vi "Read NMEA GPS GENERIC - no error - SubVI.vi"(0 "VISA resource name":refnum<visa-resource-name>="COM11", 5 "timeout (ms)":u32=10000, 7 "UTC Time Zone":i32=-5, 9 "stop":bool, 11 "error in (no error)":errorcluster, 12 "Baud Rate":dbl) -> (4 "GPS $GPRMC Data":T1 {"Course over ground (degrees)" format="%#.6g"; "Speed over ground (knots)" format="%#.6g"; "Magnetic Variation (degrees)" format="%#.6g"; "Longitude (ddmm.mmmm)" format="%#.6g"; "Lattitude (ddmm.mmmm)" format="%#.6g"}, 6 "GPS Data Valid?":bool, 10 "Stopped?":bool, 15 "error out":errorcluster)   [LabVIEW 2021]
doc: "This subVI decodes the most common NMEA-0183 sentence transmitted by GPS receivers, the $GPRMC sentence. The subvi returns time, position, ground speed, and magnetic variation. In the GPS interface configuration, use the \"NMEA OUT\" setting and set the baud rate to the standard 4800 bps setting. Connected to the computer's serial port using a PC Interface Cable, available from the GPS vendor. This subvi initializes the serial port on first call. On subsequent calls, the initialization is skipped. Always use the Stop input when stopping the VI so that the serial port connection is closed."
uses:
  <vilib>/Instr/_visa.llb/VISA Configure Serial Port (Instr).vi
panel:
  out "error out 2":errorcluster
  in  "Cluster":T1 {"Course over ground (degrees)" format="%_4g"; "Speed over ground (knots)" format="%_3g"; "Magnetic Variation (degrees)" format="%_4g"; "Longitude (ddmm.mmmm)" format="%_8g"; "Lattitude (ddmm.mmmm)" format="%_8g"}
  out "Variation\nEast/West":string
  out "Magnetic Variation \n(degrees)":dbl format="%_4g"
  out "Course over\nground (degrees)":dbl format="%_4g"
  out "Speed over \nground (knots)":dbl format="%_3g"
  out "Longitude\nEast/West":string
  out "Longitude\n(ddmm.mmmm)":dbl format="%_8g"
  out "Lattitude\nNorth/South":string
  out "Lattitude\n(ddmm.mmmm)":dbl format="%_8g"
  out "Local Time":timestamp
  out "UTC Time":timestamp
  in  "date time rec":T2
  out "Bytes read":u32
  out "String Read":string="\n"
  # "This subVI decodes the most common NMEA-0183 sentence transmitted by GPS receivers, the $GPRMC sentence. The subvi returns time, position, ground speed, and magnetic variation. In the GPS interface configuration, use the \"NMEA OUT\" setting and set the baud rate to the standard 4800 bps setting. Connected to the computer's serial port using a PC Interface Cable, available from the GPS vendor. This subvi initializes the serial port on first call. On subsequent calls, the initialization is skipped. Always use the Stop input when stopping the VI so that the serial port connection is closed."
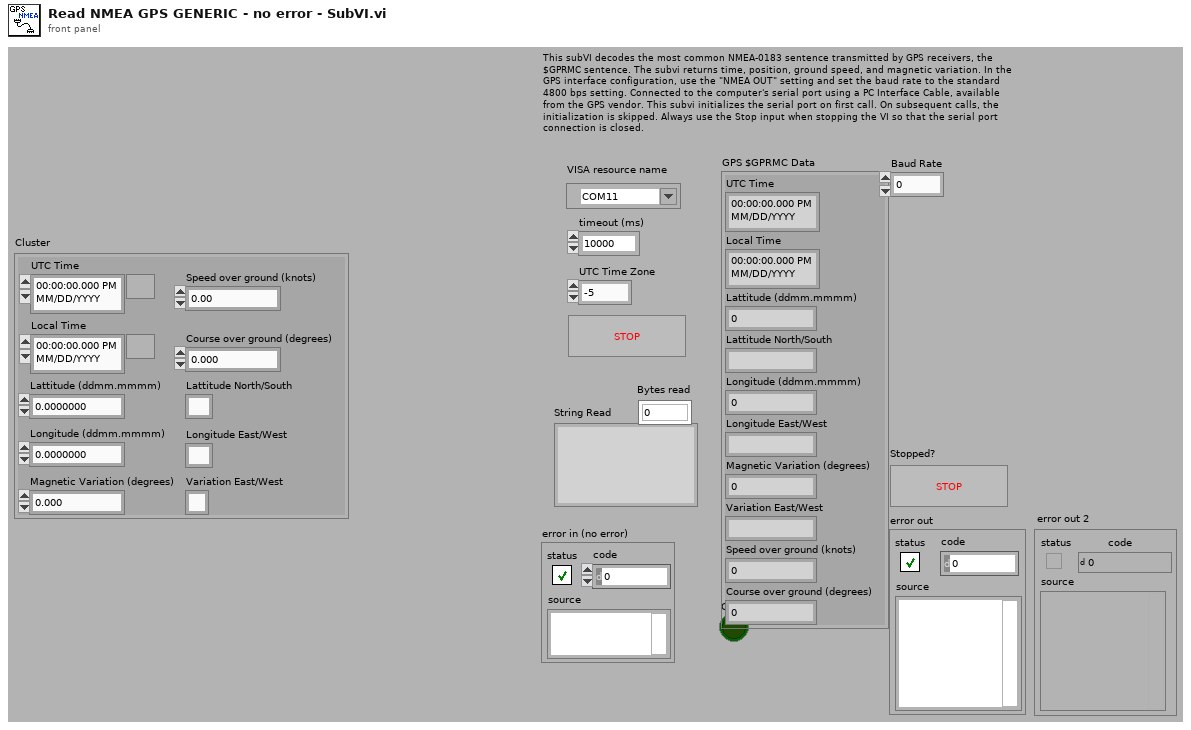
[diagram p1: front panel]
types:
  T1 = cluster{"UTC Time":timestamp, "Local Time":timestamp, "Lattitude (ddmm.mmmm)":dbl, "Lattitude North/South":string, "Longitude (ddmm.mmmm)":dbl, "Longitude East/West":string, "Magnetic Variation (degrees)":dbl, "Variation East/West":string, "Speed over ground (knots)":dbl, "Course over ground (degrees)":dbl}
  T2 = cluster{"second":i32, "minute":i32, "hour":i32, "day of month":i32, "month":i32, "year":i32, "day of week":i32, "day of year":i32, "is DST":i32}
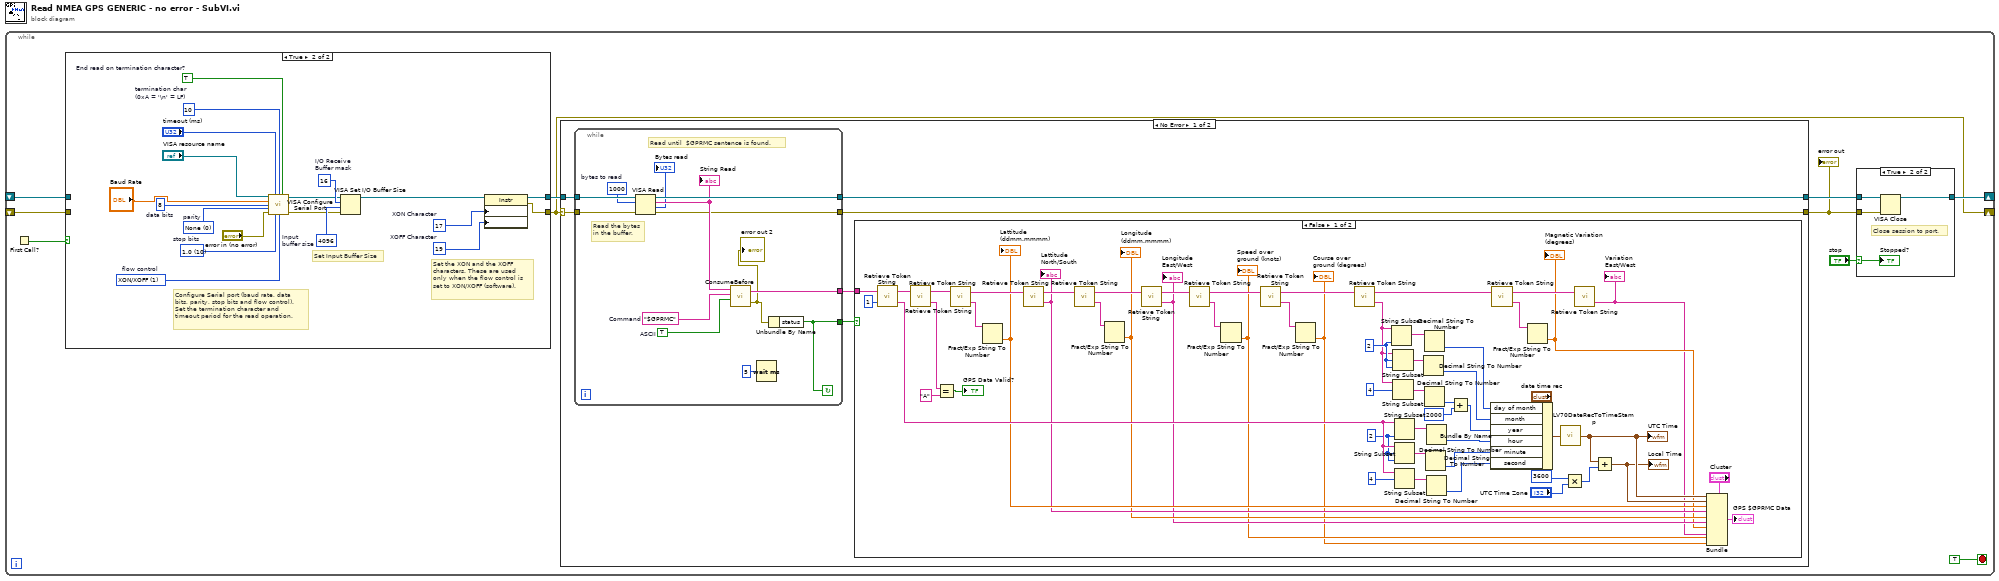
[diagram p0: block diagram]
diagram:
  n1 = while {
    shift-right: [w5] -> _
    shift-left: _ -> [w4]
    shift-right: [w3] -> _
    shift-left: _ -> [w2]
    stop <- TRUE stop-if-true
    n2 = First Call?() -> (First Call?: T/F=w8:bool)
    n3 = case shown="True" w8 {
      tunnel: [w16 w22] -> w10
      tunnel: [w15 w19] -> w3
      tunnel: w4 -> [w16 _]
      tunnel: w2 -> [w15 _]
      frame False {
      }
      frame True {
        w31 = TRUE  # End read on termination character?
        w24 = u8 19  # XOFF Character
        w25 = u8 17  # XON Character
        w29 = u32 4096  # Input buffer size
        w27 = u16 1 items=["None"=0, "XON/XOFF"=1, "RTS/CTS"=2, "DTR/DSR"=4]  # flow control
        w33 = u16 10 items=["1.0"=10, "1.5"=15, "2.0"=20]  # stop bits
        w34 = u16 0 items=["None", "Odd", "Even", "Mark", "Space"]  # parity
        w23 = u16 8  # data bits
        w28 = u8 10  # termination char (0xA = '\n' = LF)
        w30 = u16 16  # I/O Receive Buffer mask
        # "Set the XON and the XOFF\ncharacters. These are used\nonly when the flow control is\nset to XON/XOFF (software)."
        # "Configure Serial port (baud rate, data\nbits, parity, stop bits and flow control).\nSet the termination character and\ntimeout period for the read operation."
        # "Set Input Buffer Size"
        n4 = call-poly "VISA Configure Serial Port"("VISA resource name"="VISA resource name", "timeout (10sec)"="timeout (ms)", "termination char\n(0xA = '\\n' = LF)"=w28, "Enable Termination\nChar (T)"=w31, "baud rate (9600)"="Baud Rate", "data bits (8)"=w23, "parity (0:none)"=w34, "error in (no error)"="error in (no error)", "stop bits (10: 1 bit)"=w33, "flow control (0:none)"=w27) -> ("VISA resource name out"=w21:refnum<visa-resource-name>, "error out"=w20:errorcluster)  [unwired: 4 in]
        n5 = VISA Set I/O Buffer Size(VISA resource name=w21, mask (16)=w30, size (4096)=w29, error in (no error)=w20) -> (VISA resource name out=w26:refnum<visa-resource-name>)  [unwired: 1 out]
        n6 = property class="Instr"(reference=w26, "Serial Settings:Flow Control XON Character"=w25, "Serial Settings:Flow Control XOFF Character"=w24) -> (reference out=w22:refnum<visa-resource-name>, error out=w19:errorcluster)  [unwired: 1 in]
      }
    }
    n7 = case shown="No Error" w3 {
      selector: w3 -> [w39 w112]
      tunnel: w10 -> [w41 w113]
      tunnel: [w40 w113] -> w9
      tunnel: [w36 w112] -> w1
      frame No Error {
        n8 = while {
          tunnel: w41 -> [w54]
          tunnel: [w53] -> w40
          tunnel: [w43] -> w36
          tunnel: w39 -> [w52]
          tunnel: [w48] -> w38
          tunnel: [w45] -> w37
          stop <- w45 continue-if-true
          w47 = u32 1000  # bytes to read
          w51 = "$GPRMC"  # Command
          w50 = TRUE  # ASCII
          # "Read until  $GPRMC sentence is found."
          # "Read the bytes\nin the buffer."
          n9 = VISA Read(VISA resource name=w54, byte count=w47, error in (no error)=w52) -> (VISA resource name out=w53:refnum<visa-resource-name>, read buffer=w49:string, return count=→"Bytes read":u32, error out=w43:errorcluster)
          "String Read" <- w49
          n10 = call "ConsumeBefore.vi"("ASCII"=w50, "Before"=w51, "Response String In"=w49) -> ("error out"=w42:errorcluster, "Response String Out"=w48:string)  [unwired: 1 in]
          "error out 2" <- w42
          n11 = Wait (ms)(milliseconds to wait=u32 5 ("millisecond multiple")) -> ()  [unwired: 1 out]
          n12 = Unbundle By Name(w42) -> ("status"=w45:bool)
        }
        n13 = case shown="False" w37 {
          tunnel: w38 -> [w109 _]
          frame False {
            w77 = 2 ("length (rest)")
            w99 = 2 ("length (rest)")
            n14 = call "Retrieve Token String.vi"("Offset (0)"=1, "input string"=w109) -> ("token string"=w106:string, "output string"=w107:string)
            n15 = call "Retrieve Token String.vi"("input string"=w107) -> ("token string"=w111:string, "output string"=w105:string)  [unwired: 1 in]
            n16 = Equal?(x=w111, y="A") -> (x = y?=→"GPS Data Valid?":bool)
            n17 = call "Retrieve Token String.vi"("input string"=w105) -> ("token string"=w90:string, "output string"=w89:string)  [unwired: 1 in]
            n18 = Fract/Exp String To Number(string=w90) -> (number=w64:dbl)  [unwired: 3 in, 1 out]
            "Lattitude\n(ddmm.mmmm)" <- w64
            n19 = call "Retrieve Token String.vi"("input string"=w89) -> ("token string"=w63:string, "output string"=w88:string)  [unwired: 1 in]
            "Lattitude\nNorth/South" <- w63
            n20 = call "Retrieve Token String.vi"("input string"=w88) -> ("token string"=w87:string, "output string"=w86:string)  [unwired: 1 in]
            n21 = Fract/Exp String To Number(string=w87) -> (number=w62:dbl)  [unwired: 3 in, 1 out]
            "Longitude\n(ddmm.mmmm)" <- w62
            n22 = call "Retrieve Token String.vi"("input string"=w86) -> ("token string"=w61:string, "output string"=w85:string)  [unwired: 1 in]
            "Longitude\nEast/West" <- w61
            n23 = call "Retrieve Token String.vi"("input string"=w85) -> ("token string"=w84:string, "output string"=w83:string)  [unwired: 1 in]
            n24 = Fract/Exp String To Number(string=w84) -> (number=w58:dbl)  [unwired: 3 in, 1 out]
            "Speed over \nground (knots)" <- w58
            n25 = call "Retrieve Token String.vi"("input string"=w83) -> ("token string"=w82:string, "output string"=w81:string)  [unwired: 1 in]
            n26 = Fract/Exp String To Number(string=w82) -> (number=w57:dbl)  [unwired: 3 in, 1 out]
            "Course over\nground (degrees)" <- w57
            n27 = call "Retrieve Token String.vi"("input string"=w81) -> ("token string"=w75:string, "output string"=w69:string)  [unwired: 1 in]
            n28 = String Subset(string=w75, length (rest)=w77) -> (substring=w76:string)  [unwired: 1 in]
            n29 = String Subset(string=w75, offset (0)=w77, length (rest)=w77) -> (substring=w78:string)
            n30 = String Subset(string=w75, offset (0)=4) -> (substring=w80:string)  [unwired: 1 in]
            n31 = String Subset(string=w106, length (rest)=w99) -> (substring=w103:string)  [unwired: 1 in]
            n32 = String Subset(string=w106, offset (0)=w99, length (rest)=w99) -> (substring=w97:string)
            n33 = String Subset(string=w106, offset (0)=4) -> (substring=w95:string)  [unwired: 1 in]
            n34 = Decimal String To Number(string=w78) -> (number=w73:i32)  [unwired: 2 in, 1 out]
            n35 = Decimal String To Number(string=w76) -> (number=w74:i32)  [unwired: 2 in, 1 out]
            n36 = Decimal String To Number(string=w80) -> (number=w72:i32)  [unwired: 2 in, 1 out]
            n37 = Decimal String To Number(string=w97) -> (number=w98:i32)  [unwired: 2 in, 1 out]
            n38 = Decimal String To Number(string=w103) -> (number=w100:i32)  [unwired: 2 in, 1 out]
            n39 = Decimal String To Number(string=w95) -> (number=w94:i32)  [unwired: 2 in, 1 out]
            n40 = Add(x=w72, y=2000) -> (x+y=w70:i32)
            n41 = Bundle By Name(cluster="date time rec", "day of month"=w74, "month"=w73, "year"=w70, "hour"=w100, "minute"=w98, "second"=w94) -> (w102:T2)
            n42 = call "Retrieve Token String.vi"("input string"=w69) -> ("token string"=w68:string, "output string"=w67:string)  [unwired: 1 in]
            n43 = Fract/Exp String To Number(string=w68) -> (number=w60:dbl)  [unwired: 3 in, 1 out]
            "Magnetic Variation \n(degrees)" <- w60
            n44 = call <vilib>:"LV70DateRecToTimeStamp.vi"("date time rec"=w102) -> ("Time Stamp"=w66:timestamp)
            "UTC Time" <- w66
            n45 = Multiply(x=3600 ("number"), y="UTC Time Zone") -> (x*y=w91:i32)
            n46 = call "Retrieve Token String.vi"("input string"=w67) -> ("token string"=w59:string)  [unwired: 1 in, 1 out]
            "Variation\nEast/West" <- w59
            n47 = Add(x=w66, y=w91) -> (x+y=w65:timestamp)
            "Local Time" <- w65
            n48 = Bundle(cluster="Cluster", "UTC Time"=w66, "Local Time"=w65, "Lattitude (ddmm.mmmm)"=w64, "Lattitude North/South"=w63, "Longitude (ddmm.mmmm)"=w62, "Longitude East/West"=w61, "Magnetic Variation (degrees)"=w60, "Variation East/West"=w59, "Speed over ground (knots)"=w58, "Course over ground (degrees)"=w57) -> (→"GPS $GPRMC Data":T1)
          }
          frame True {
          }
        }
      }
      frame Error {
      }
    }
    "error out" <- w1
    n49 = case shown="True" "stop" {
      selector: "stop" -> [_ w12]
      tunnel: w9 -> [w11 w13]
      tunnel: w1 -> [_ w14]
      tunnel: [w11 w13] -> w5
      frame False {
      }
      frame True {
        # "Close session to port."
        n50 = VISA Close(VISA resource name=w13, error in (no error)=w14) -> ()  [unwired: 1 out]
        "Stopped?" <- w12
      }
    }
  }
